vi "Voltage_Difference.vi"(8 "error in (no error)":errorcluster, 9 "Sample":dbl format="%#_13g", 11 "Desired Voltage":dbl format="%_7g") -> (0 "error out":errorcluster)   [LabVIEW 2020]
uses:
  <vilib>/express/express arith-compare/Formula/XNode/ExpressFormulaBlockNode.xnode
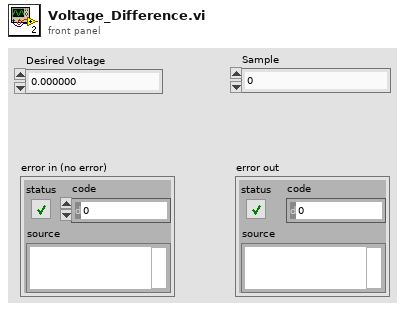
[diagram p1: front panel]
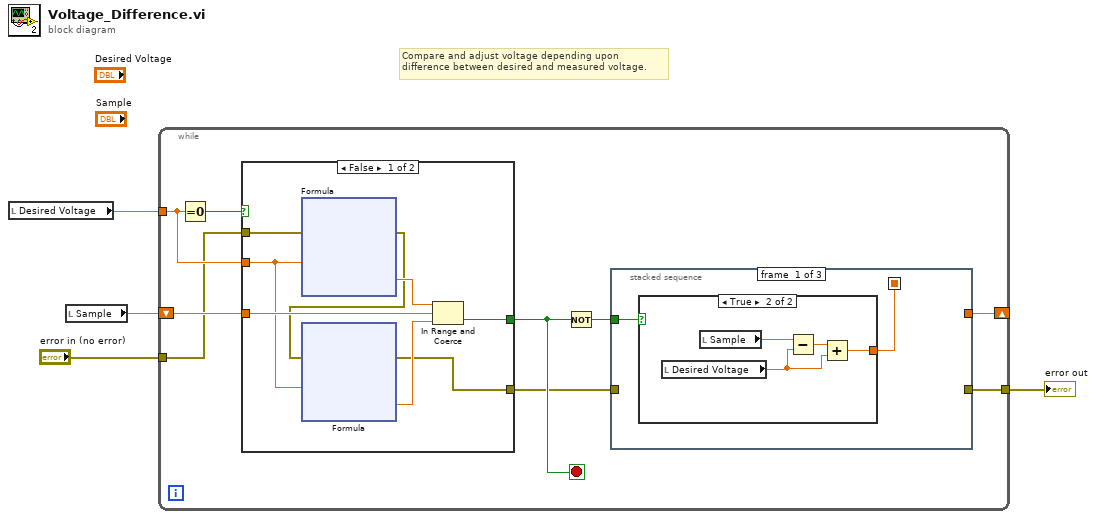
[diagram p0: block diagram]
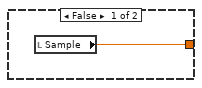
[diagram p2: hidden frame]
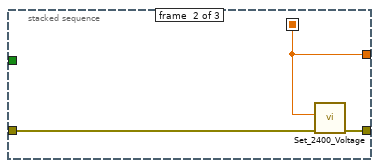
[diagram p3: hidden frame]
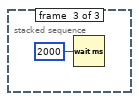
[diagram p4: hidden frame]
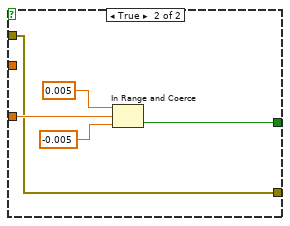
[diagram p5: hidden frame]
diagram:
  # "Compare and adjust voltage depending upon\ndifference between desired and measured voltage."
  n1 = local read "Desired Voltage"() -> (w4:dbl)
  n2 = local read "Sample"() -> (w3:dbl)
  n3 = while {
    tunnel: w4 -> [w12]
    tunnel: "error in (no error)" -> [w9]
    tunnel: [w6] -> w1
    shift-right: [w5] -> _
    shift-left: w3 -> [w11]
    stop <- w8 stop-if-true
    n4 = Equal To 0?(x=w12) -> (x = 0?=w13:bool)
    n5 = case shown="False" w13 {
      tunnel: w11 -> [w30 w51]
      tunnel: w12 -> [w29 _]
      tunnel: [w28 w50] -> w8
      tunnel: w9 -> [w27 w49]
      tunnel: [w25 w49] -> w7
      frame False {
        n6 = xnode "Formula"("X1"=w29, "error in (no error)"=w27) -> ("Result"=w32:dbl, "error out"=w26:errorcluster)
        n7 = xnode "Formula"("X1"=w29, "error in (no error)"=w26) -> ("Result"=w31:dbl, "error out"=w25:errorcluster)
        n8 = In Range and Coerce(upper limit=w32, x=w30, lower limit=w31) -> (In Range?=w28:bool)  [unwired: 1 out]
      }
      frame True {
        n9 = In Range and Coerce(upper limit=0.005, x=w51, lower limit=-0.005) -> (In Range?=w50:bool)  [unwired: 1 out]
      }
    }
    n10 = Not(x=w8) -> (.not. x?=w10:bool)
    n11 = stacked-sequence {
      seq-local: [w14 _ _] -> [_ w21 _]
      tunnel: w10 -> [w15 _ _]
      tunnel: w7 -> [_ w23 _]
      tunnel: [_ w22 _] -> w6
      tunnel: [_ w21 _] -> w5
      frame #0 {
        n12 = case shown="True" w15 {
          tunnel: [w16 w17] -> w14
          frame False {
            n13 = local read "Sample"() -> (w16:dbl)
          }
          frame True {
            n14 = local read "Desired Voltage"() -> (w18:dbl)
            n15 = local read "Sample"() -> (w20:dbl)
            n16 = Subtract(x=w20, y=w18) -> (x-y=w19:dbl)
            n17 = Add(x=w19, y=w18) -> (x+y=w17:dbl)
          }
        }
      }
      frame #1 {
        n18 = call "Set_2400_Voltage.vi"("error in"=w23, "Voltage"=w21) -> ("error out"=w22:errorcluster)  [unwired: 8 in]
      }
      frame #2 {
        n19 = Wait (ms)(milliseconds to wait=u32 2000) -> ()  [unwired: 1 out]
      }
    }
  }
  "error out" <- w1
